vi "PQrequestCancel.vi"(8 "error in (no error)":errorcluster, 11 "conn":u64) -> (0 "error out":errorcluster, 2 "PQrequestCancel":i64, 3 "conn_out":u64)   [LabVIEW 2019, in "libpqlv64.lvlib"]
uses:
  libpqlv64.lvlib
  libpq.dll
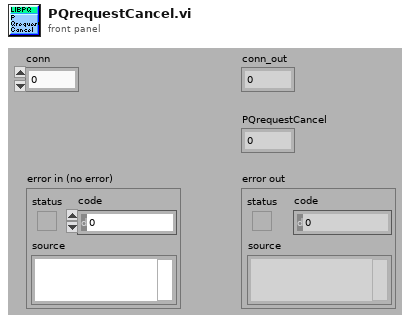
[diagram p1: front panel]
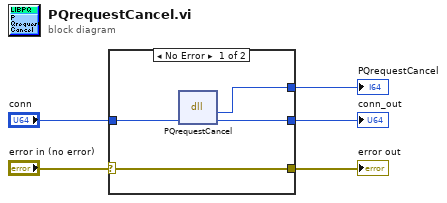
[diagram p0: block diagram]
diagram:
  n1 = case shown="No Error" "error in (no error)" {
    selector: "error in (no error)" -> [w9 w11]
    tunnel: [w9 w11] -> w4
    tunnel: [w8 _] -> w3
    tunnel: [w7 w10] -> w2
    tunnel: "conn" -> [w6 w10]
    frame No Error {
      n2 = dll-call lib="libpq.*" fn="PQrequestCancel"("conn"=w6) -> ("PQrequestCancel"=w8:i64, "conn"=w7:u64)  [unwired: 3 in, 2 out]
    }
    frame Error {
    }
  }
  "PQrequestCancel" <- w3
  "error out" <- w4
  "conn_out" <- w2
